vi "3D_Traverse_move_manual.vi"() -> ()   [LabVIEW 2011]
uses:
  Controls/Tunnel_Coordinates.ctl
  Trav_mode.ctl
  Controls/User_Specific_mode.ctl
  Globals/Constants_global.vi
panel:
  out "Current Traverse 2":string
  out "Current Traverse":string
  in  "Work in Tunnel Coordinates":T1
  in  "Traverse":u16(ring) items=["Aero_Enclosure", "Aero_Sting", "Aero_ThroughWall", "Aero_Tunnel", "Dummy", "PIV_Traverse"]
  in  "stop":bool
  in  "Increment":dbl=10.0
  in  "Z-":bool
  in  "Z+":bool
  in  "Y+":bool
  in  "Y-":bool
  in  "X+":bool
  in  "X-":bool
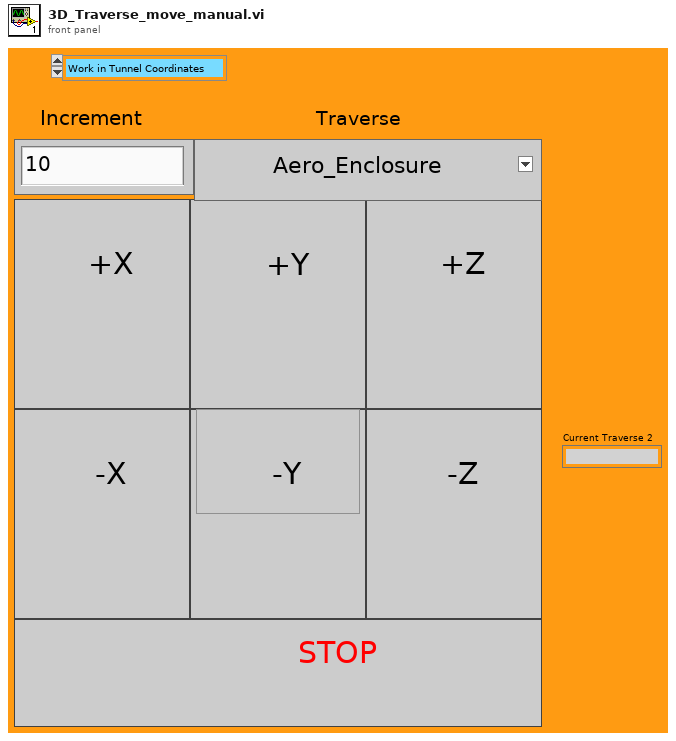
[diagram p1: front panel]
types:
  T1 = typedef "Tunnel_Coordinates.ctl" = enum16{"Work in Tunnel Coordinates", "Work in Model Coordinates"}
  T2 = typedef "User_Specific_mode.ctl" = enum16{"Check VI only", "Run VI"}
  T3 = typedef "Trav_mode.ctl" = enum16{"Move traverse", "Read traverse position", "Teach Position"}
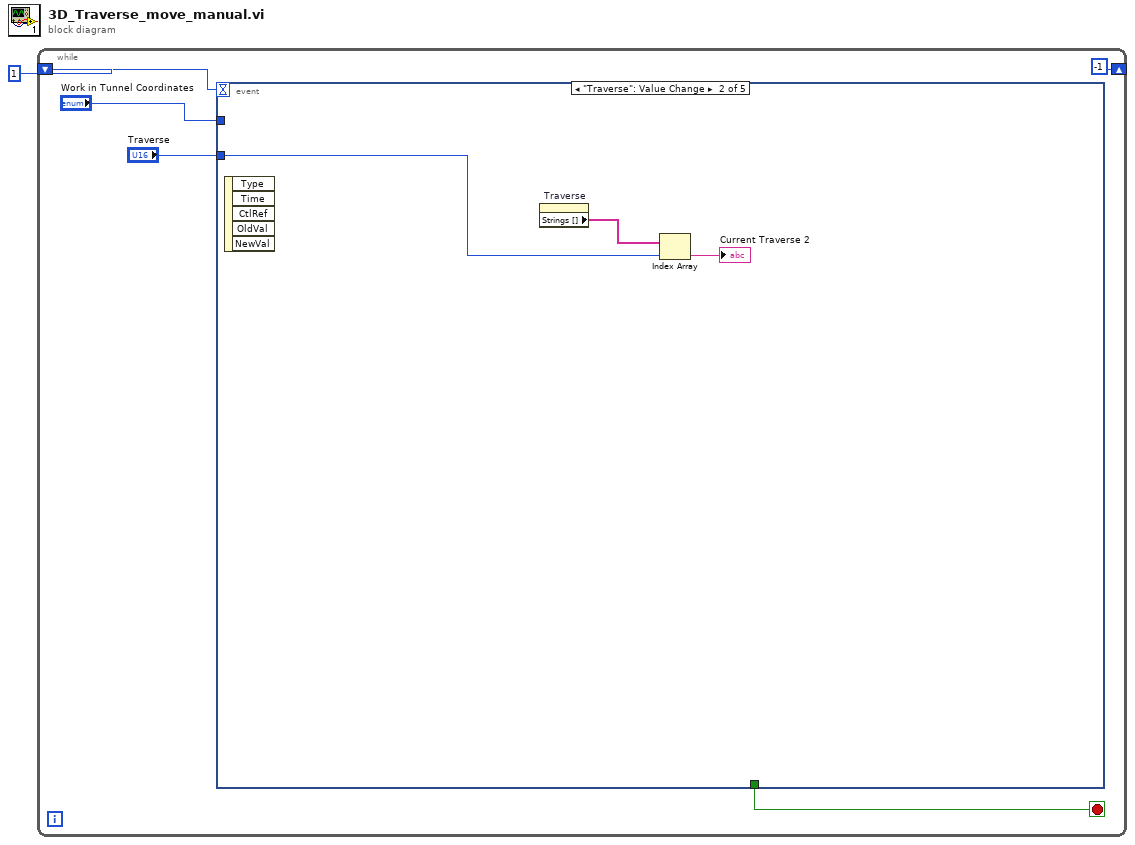
[diagram p0: block diagram]
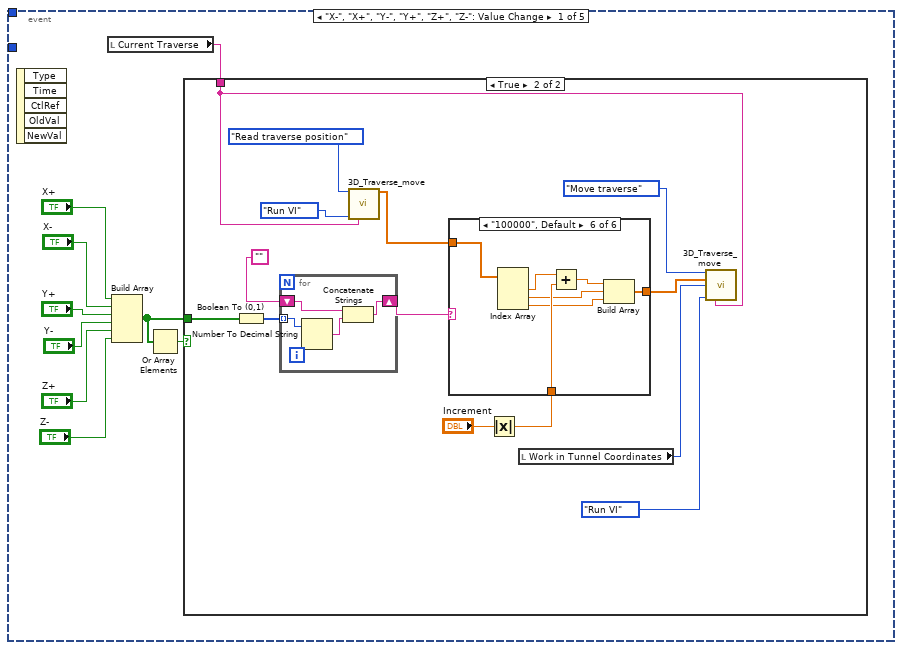
[diagram p2: hidden frame]
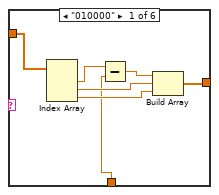
[diagram p4: hidden frame]
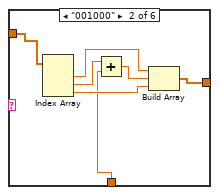
[diagram p5: hidden frame]
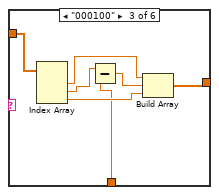
[diagram p6: hidden frame]
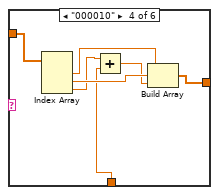
[diagram p7: hidden frame]
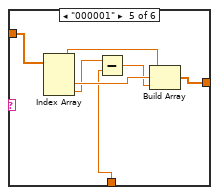
[diagram p8: hidden frame]
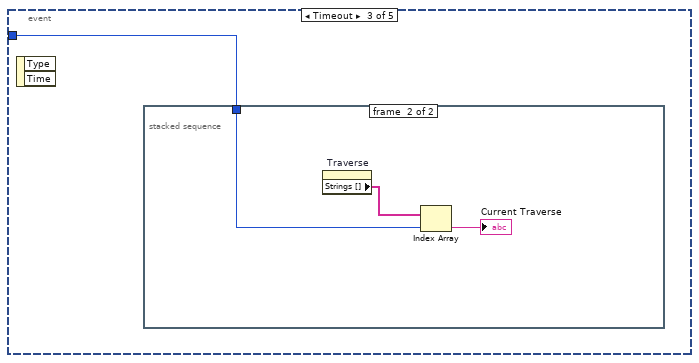
[diagram p9: hidden frame]
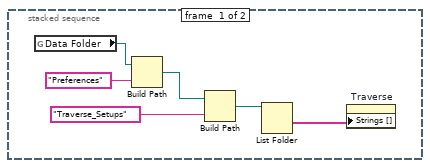
[diagram p10: hidden frame]
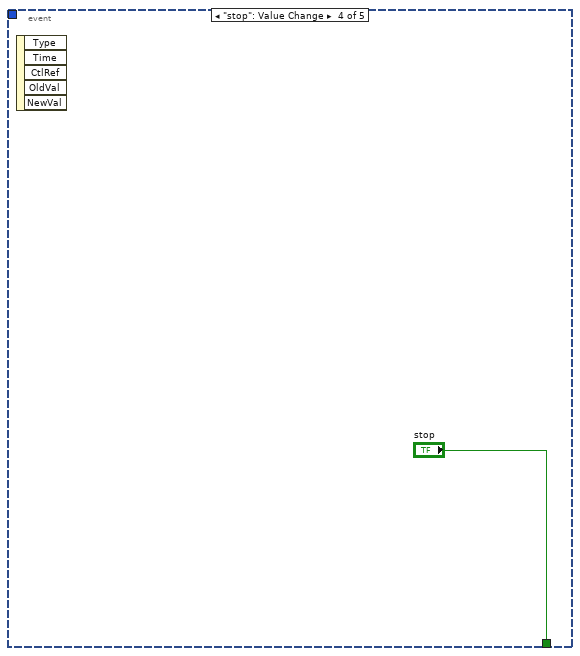
[diagram p11: hidden frame]
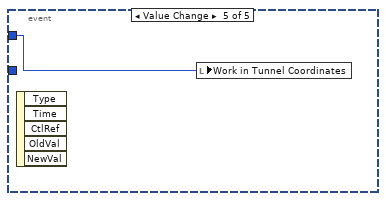
[diagram p12: hidden frame]
diagram:
  n1 = while {
    shift-right: [-1] -> _
    shift-left: 1 -> [w2]
    stop <- w6 stop-if-true
    n2 = event shown="[1] \"Traverse\": Value Change" {
      selector: _ -> [_ _ _ _ _]
      dyn-events: _ -> [_ _ _ _ _]
      timeout: w2 -> [_ _ _ _ _]
      tunnel: [_ _ _ "stop" _] -> w6
      tunnel: "Traverse" -> [_ w76 w79 _ _]
      tunnel: "Work in Tunnel Coordinates" -> [_ _ _ _ w90]
      event "X-", "X+", "Y-", "Y+", "Z+", "Z-": Value Change {
        n3 = event-data() -> ()  [unwired: 1 in, 5 out]
        n4 = local read "Current Traverse"() -> (w7:string)
        n5 = Build Array("X+", "X-", "Y+", "Y-", "Z+", "Z-") -> (w8:bool[])
        n6 = Or Array Elements(Boolean array=w8) -> (logical OR=w9:bool)
        n7 = case shown="True" w9 {
          tunnel: w8 -> [_ w20]
          tunnel: w7 -> [_ w16]
          frame False {
          }
          frame True {
            n8 = Boolean To (0,1)(Boolean=w20) -> (0, 1=w28:i16[])
            n9 = for {
              shift-right: [w32] -> w27
              shift-left: "" -> [w33]
              tunnel: w28 -> [w31] mode=indexing
              n10 = Number To Decimal String(number=w31) -> (decimal integer string=w30:string)  [unwired: 1 in]
              n11 = Concatenate Strings(w33, w30) -> (w32:string)
            }
            n12 = call "3D_Traverse_move.vi"("Mode"=Trav_mode."Read traverse position", "Simulate/Run"=User_Specific_mode."Run VI", "Traverse name"=w16) -> ("Trav Position achieved"=w17:dbl[])  [unwired: 10 in, 2 out]
            n13 = Absolute Value(x="Increment") -> (abs(x)=w25:dbl)
            n14 = case shown="\"100000\", Default" w27 {
              tunnel: w17 -> [w34 w46 w50 w60 w67 w75]
              tunnel: w25 -> [w35 w45 w49 w56 w66 w73]
              tunnel: [w36 w41 w48 w55 w62 w69] -> w24
              frame "010000" {
                n15 = Index Array(array=w34) -> (element #1=w40:dbl, element #2=w38:dbl, element #3=w37:dbl)  [unwired: 3 in]
                n16 = Subtract(x=w40, y=w35) -> (x-y=w39:dbl)
                n17 = Build Array(w39, w38, w37) -> (w36:dbl[])
              }
              frame "001000" {
                n18 = Index Array(array=w46) -> (element #1=w43:dbl, element #2=w42:dbl, element #3=w47:dbl)  [unwired: 3 in]
                n19 = Add(x=w42, y=w45) -> (x+y=w44:dbl)
                n20 = Build Array(w43, w44, w47) -> (w41:dbl[])
              }
              frame "000100" {
                n21 = Index Array(array=w50) -> (element #1=w51:dbl, element #2=w53:dbl, element #3=w54:dbl)  [unwired: 3 in]
                n22 = Subtract(x=w53, y=w49) -> (x-y=w52:dbl)
                n23 = Build Array(w51, w52, w54) -> (w48:dbl[])
              }
              frame "000010" {
                n24 = Index Array(array=w60) -> (element #1=w57:dbl, element #2=w61:dbl, element #3=w59:dbl)  [unwired: 3 in]
                n25 = Add(x=w59, y=w56) -> (x+y=w58:dbl)
                n26 = Build Array(w57, w61, w58) -> (w55:dbl[])
              }
              frame "000001" {
                n27 = Index Array(array=w67) -> (element #1=w63:dbl, element #2=w68:dbl, element #3=w65:dbl)  [unwired: 3 in]
                n28 = Subtract(x=w65, y=w66) -> (x-y=w64:dbl)
                n29 = Build Array(w63, w68, w64) -> (w62:dbl[])
              }
              frame "100000", Default {
                n30 = Index Array(array=w75) -> (element #1=w74:dbl, element #2=w71:dbl, element #3=w70:dbl)  [unwired: 3 in]
                n31 = Add(x=w74, y=w73) -> (x+y=w72:dbl)
                n32 = Build Array(w72, w71, w70) -> (w69:dbl[])
              }
            }
            n33 = local read "Work in Tunnel Coordinates"() -> (w22:T1)
            n34 = call "3D_Traverse_move.vi"("Mode"=Trav_mode."Move traverse", "Position"=w24, "Work in Tunnel Coordinates"=w22, "Simulate/Run"=User_Specific_mode."Run VI", "Traverse name"=w16) -> ()  [unwired: 8 in, 3 out]
          }
        }
      }
      event "Traverse": Value Change {
        n35 = event-data() -> ()  [unwired: 1 in, 5 out]
        n36 = property on="Traverse" class="Ring (strict)"() -> ("Strings []"=w77:string[])  [unwired: 2 in, 2 out]
        n37 = Index Array(array=w77, index=w76) -> (element=→"Current Traverse 2":string)
      }
      event Timeout {
        n38 = event-data() -> ()  [unwired: 1 in, 2 out]
        n39 = stacked-sequence {
          tunnel: w79 -> [_ w87]
          frame #0 {
            n40 = global read "Constants_global.vi" "Data Folder"() -> (w82:path)
            n41 = Build Path(base path=w82, name or relative path="Preferences") -> (appended path=w84:path)
            n42 = Build Path(base path=w84, name or relative path="Traverse_Setups") -> (appended path=w85:path)
            n43 = List Folder(path=w85) -> (folder names=w80:string[])  [unwired: 1 in, 5 out]
            n44 = property on="Traverse" class="Ring (strict)"("Strings []"=w80) -> ()  [unwired: 2 in, 2 out]
          }
          frame #1 {
            n45 = property on="Traverse" class="Ring (strict)"() -> ("Strings []"=w88:string[])  [unwired: 2 in, 2 out]
            n46 = Index Array(array=w88, index=w87) -> (element=→"Current Traverse":string)
          }
        }
      }
      event "stop": Value Change {
        n47 = event-data() -> ()  [unwired: 1 in, 5 out]
      }
      event Value Change {
        n48 = event-data() -> ()  [unwired: 1 in, 5 out]
        n49 = local write "Work in Tunnel Coordinates"(w90) -> ()
      }
    }
  }
